vi "método euler.vi"() -> ()   [LabVIEW 2018]
uses:
  <vilib>/express/express arith-compare/Formula/XNode/ExpressFormulaBlockNode.xnode
panel:
  in  "stop":bool
  in  "y_0":dbl
  out "XY Graph":cluster{"Y":dbl[], "Y":dbl[]}[](graph)
  out "h":dbl
  in  "número de intervalos":dbl
  in  "Condición final b":dbl
  in  "Condición inicial a":dbl
  # "x^2"
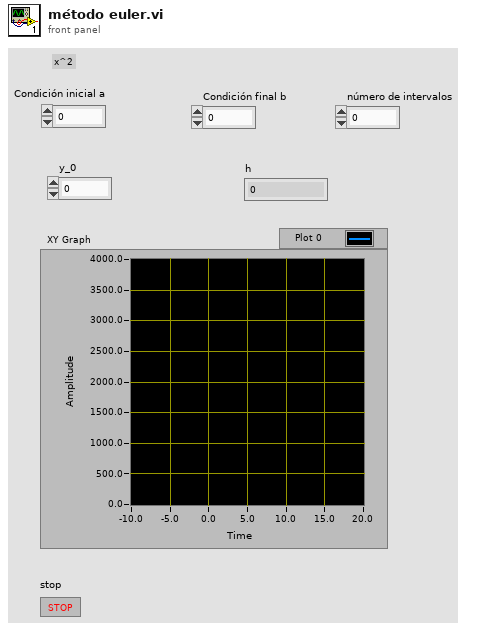
[diagram p1: front panel]
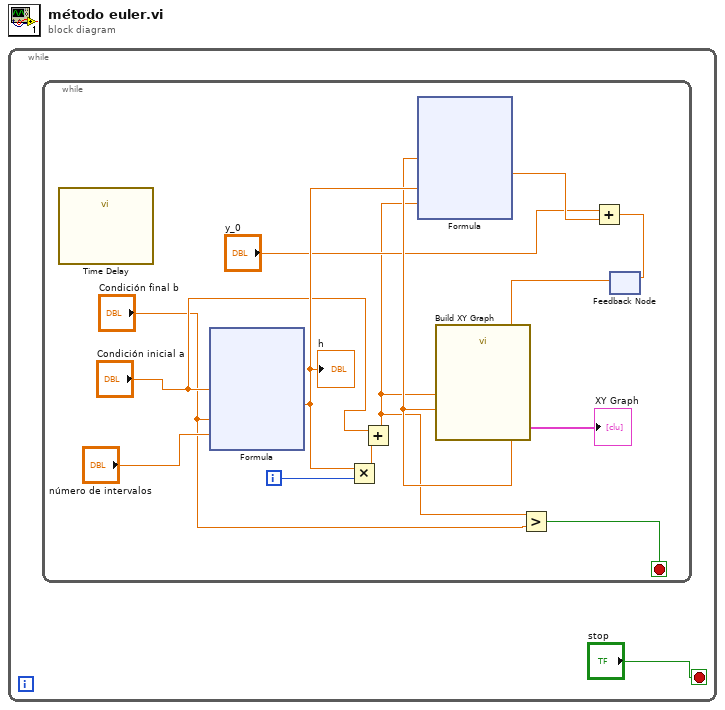
[diagram p0: block diagram]
diagram:
  n1 = while {
    stop <- "stop" stop-if-true
    n2 = while {
      i -> [w11]
      stop <- w2 stop-if-true
      n3 = call "Time Delay"() -> ()  [unwired: 11 in, 1 out]
      n4 = xnode "Formula"("a"="Condición inicial a", "b"="Condición final b", "n"="número de intervalos") -> ("Result"=w10:dbl)  [unwired: 1 in, 1 out]
      "h" <- w10
      n5 = Multiply(x=w10, y=w11) -> (x*y=w9:dbl)
      n6 = Add(x="Condición inicial a", y=w9) -> (x+y=w4:dbl)
      n7 = Greater?(x=w4, y="Condición final b") -> (0:w2:bool)
      n8 = feedback #1() -> (w7:dbl)  [unwired: 1 in]
      n9 = xnode "Formula"("y_0"=w7, "h"=w10, "x"=w4) -> ("Result"=w13:dbl)  [unwired: 1 in, 1 out]
      n10 = call "Build XY Graph"("Y Input"=w7, "X Input"=w4) -> ("XY Graph"=→"XY Graph":cluster{"X":dbl[], "Y":dbl[]}[])  [unwired: 8 in, 1 out]
      n11 = Add(x="y_0", y=w13) -> (x+y=w12:dbl)
      n12 = feedback-in #1(w12) -> ()
    }
  }
